vi "Line Output.vi"(8 "error in (no error)":errorcluster, 9 "position (0, 0)":cluster{"row":i8, "column":i8}, 10 "character codes":u8[](array[numeric])=[48, 49, 50, 51, 52, 53, 54, 55, 56, 57], 11 "cluster of private data in":T1={"FPGA VI Reference"=refnum, "device index"=0, "screen size"=enum."8x1", "font size"=enum."5x8", "auto wrap"=FALSE, "alignment"=enum."None", "number of line"=enum."2 lines", "shift 0"=0, "entry mode 0"=enum."increment & no shift", "shift 1"=0, "entry mode 1"=enum."increment & no shift"}) -> (0 "error out":errorcluster, 1 "current position":cluster{"row":i8, "column":i8}, 3 "cluster of private data out":T1={"FPGA VI Reference"=refnum, "device index"=0, "screen size"=enum."8x1", "font size"=enum."5x8", "auto wrap"=FALSE, "alignment"=enum."None", "number of line"=enum."2 lines", "shift 0"=0, "entry mode 0"=enum."increment & no shift", "shift 1"=0, "entry mode 1"=enum."increment & no shift"})   [LabVIEW 2017, in "HD44780.lvclass"]
uses:
  HD44780.lvclass
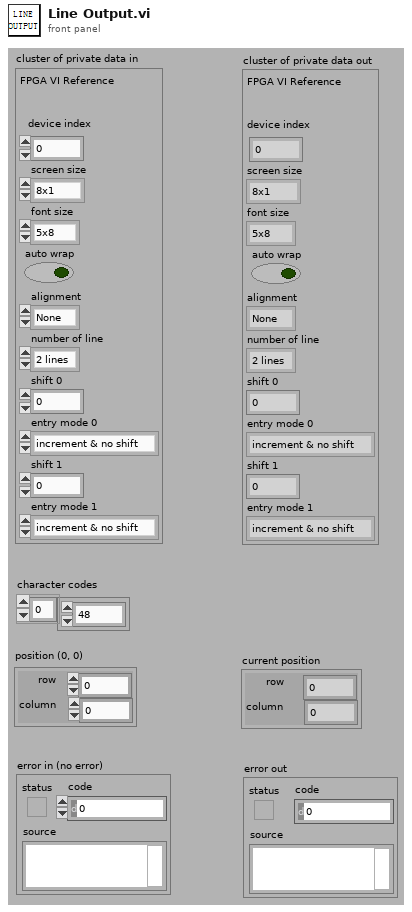
[diagram p1: front panel]
types:
  T1 = cluster{"FPGA VI Reference":refnum<k20>, "device index":i8, "screen size":enum8{"8x1", "8x2", "12x4", "16x1", "16x2", "16x4", "20x1", "20x2", "20x4", "24x1", "24x2", "40x2", "40x4"}, "font size":enum8{"5x8", "5x10"}, "auto wrap":bool, "alignment":enum16{"None", "Left", "Center", "Right"}, "number of line":enum8{"1 line", "2 lines"}, "shift 0":i8, "entry mode 0":enum8{"increment & no shift", "increment & shift", "decrement & no shift", "decrement & shift"}, "shift 1":i8, "entry mode 1":enum8{"increment & no shift", "increment & shift", "decrement & no shift", "decrement & shift"}}
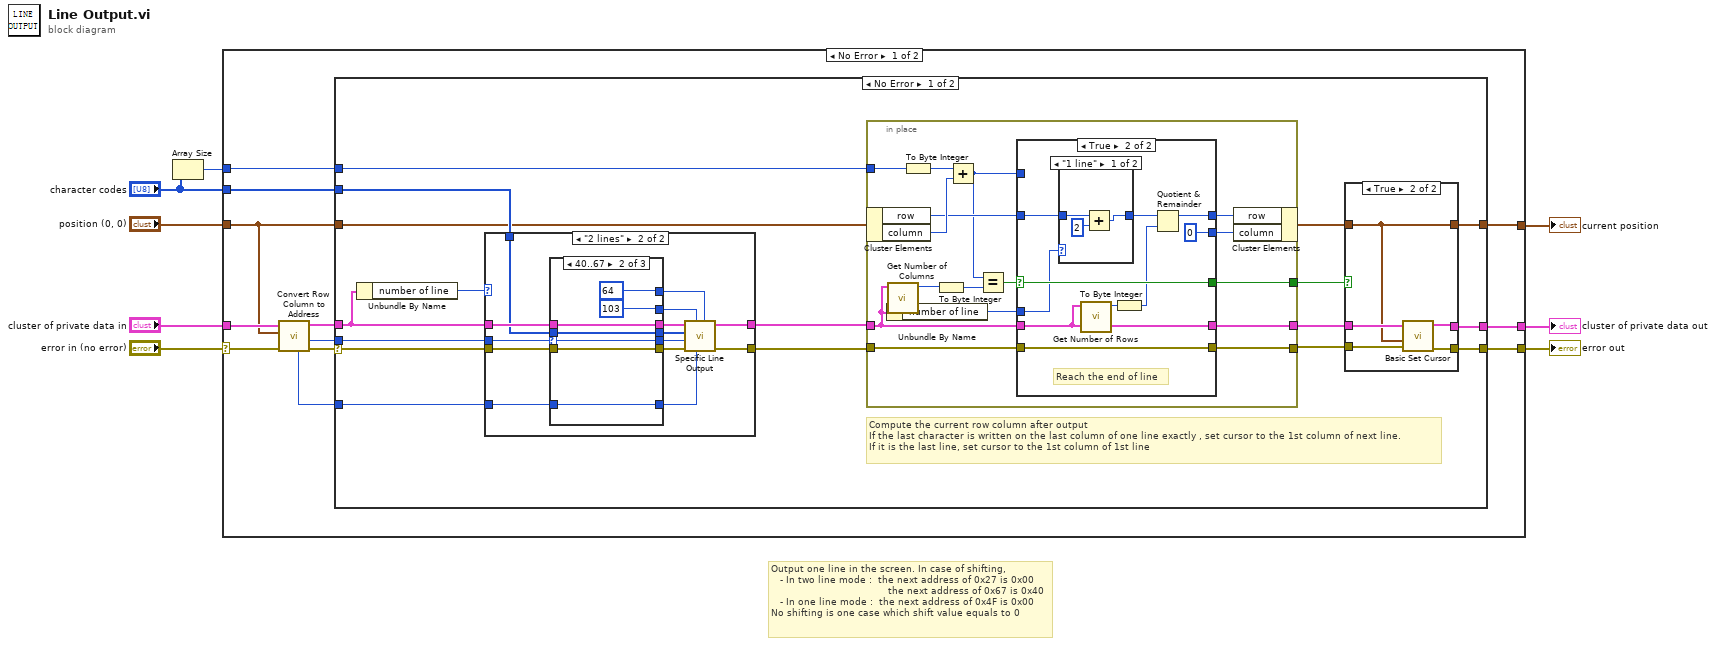
[diagram p0: block diagram]
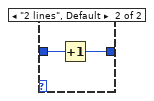
[diagram p4: hidden frame]
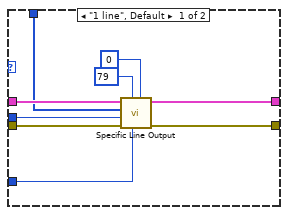
[diagram p5: hidden frame]
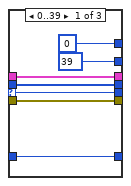
[diagram p6: hidden frame]
diagram:
  # "Output one line in the screen. In case of shifting,\n   - In two line mode :  the next address of 0x27 is 0x00\n                                       the next address of 0x67 is 0x40\n   - In one line mode :  the next address of 0x4F is 0x00\nNo shifting is one case which shift value equals to 0"
  n1 = Array Size(array="character codes") -> (size(s)=w5:i32)
  n2 = case shown="No Error" "error in (no error)" {
    selector: "error in (no error)" -> [w16 w129]
    tunnel: [w12 w129] -> w1
    tunnel: "character codes" -> [w19 _]
    tunnel: "position (0, 0)" -> [w14 w127]
    tunnel: "cluster of private data in" -> [w17 w128]
    tunnel: [w13 w128] -> w2
    tunnel: w5 -> [w15 _]
    tunnel: [w11 w127] -> w3
    frame No Error {
      n3 = call "Convert Row Column to Address.vi"("error in (no error)"=w16, "cursor position"=w14, "cluster of private data in"=w17) -> ("error out"=w9:errorcluster, "address"=w10:u8, "cluster of private data out"=w20:T1, "chip select"=w18:enum16{"1st chip", "2nd chip"})  [unwired: 5 in]
      n4 = case shown="No Error" w9 {
        selector: w9 -> [w21 w124]
        tunnel: w20 -> [w37 w125]
        tunnel: w19 -> [w35 _]
        tunnel: w18 -> [w34 _]
        tunnel: w15 -> [w31 _]
        tunnel: w14 -> [w30 w126]
        tunnel: [w29 w125] -> w13
        tunnel: [w28 w124] -> w12
        tunnel: [w27 w126] -> w11
        tunnel: w10 -> [w26 _]
        frame No Error {
          # "Compute the current row column after output\nIf the last character is written on the last column of one line exactly , set cursor to the 1st column of next line.\nIf it is the last line, set cursor to the 1st column of 1st line"
          n5 = Unbundle By Name(w37) -> ("number of line"=w36:enum8{"1 line", "2 lines"})
          n6 = case shown="\"2 lines\"" w36 {
            tunnel: w37 -> [w88 w104]
            tunnel: w35 -> [w87 w102]
            tunnel: w34 -> [w84 w101]
            tunnel: w26 -> [w86 w100]
            tunnel: w21 -> [w85 w103]
            tunnel: [w83 w96] -> w32
            tunnel: [w82 w97] -> w33
            frame "1 line", Default {
              n7 = call "Specific Line Output.vi"("turn over address"=u8 0, "chip select"=w84, "end address"=u8 79, "error in (no error)"=w85, "start address"=w86, "character codes"=w87, "cluster of private data in"=w88) -> ("error out"=w83:errorcluster, "cluster of private data out"=w82:T1)  [unwired: 3 in]
            }
            frame "2 lines" {
              n8 = case shown="40..67" w100 {
                selector: w100 -> [w105 w113 w119]
                tunnel: w104 -> [w109 w118 w123]
                tunnel: w103 -> [w107 w117 w120]
                tunnel: w102 -> [w108 w114 w122]
                tunnel: w101 -> [w106 w112 w121]
                tunnel: [w109 w118 w123] -> w99
                tunnel: [w107 w117 w120] -> w98
                tunnel: [u8 0 u8 64 _] -> w95
                tunnel: [u8 39 u8 103 _] -> w94
                tunnel: [w108 w114 w122] -> w93
                tunnel: [w105 w113 w119] -> w92
                tunnel: [w106 w112 w121] -> w91
                frame 0..39 {
                }
                frame 64..103 {
                }
                frame Default {
                }
              }
              n9 = call "Specific Line Output.vi"("turn over address"=w95, "chip select"=w91, "end address"=w94, "error in (no error)"=w98, "start address"=w92, "character codes"=w93, "cluster of private data in"=w99) -> ("error out"=w96:errorcluster, "cluster of private data out"=w97:T1)  [unwired: 3 in]
            }
          }
          n10 = in-place {
            in-place-border: w31 -> [w60]
            in-place-border: w33 -> [w47]
            in-place-border: w32 -> [w50]
            in-place-border: [w49] -> w24
            in-place-border: [w51] -> w23
            in-place-border: [w48] -> w25
            n11 = in-place-cluster #1(w30) -> ("row"=w56:i8, "column"=w61:i8)
            n12 = Unbundle By Name(w47) -> ("number of line"=w46:enum8{"1 line", "2 lines"})
            n13 = call "Get Number of Columns.vi"("cluster of private data in"=w47) -> ("column number"=w52:u8)  [unwired: 10 in]
            n14 = To Byte Integer(number=w60) -> (8bit integer=w59:i8)
            n15 = To Byte Integer(number=w52) -> (8bit integer=w58:i8)
            n16 = Add(x=w59, y=w61) -> (x+y=w54:i8)
            n17 = Equal?(x=w54, y=w58) -> (x = y?=w57:bool)
            n18 = case shown="True" w57 {
              selector: w57 -> [w62 w75]
              tunnel: w56 -> [w66 w72]
              tunnel: [w66 w67] -> w55
              tunnel: w54 -> [w65 _]
              tunnel: [w65 i8 0] -> w53
              tunnel: w47 -> [w64 w71]
              tunnel: [w64 w71] -> w51
              tunnel: w50 -> [w63 w74]
              tunnel: [w63 w74] -> w49
              tunnel: [w62 w75] -> w48
              tunnel: w46 -> [_ w73]
              frame False {
              }
              frame True {
                # "Reach the end of line"
                n19 = case shown="\"1 line\"" w73 {
                  tunnel: w72 -> [w79 w81]
                  tunnel: [w77 w80] -> w69
                  frame "1 line" {
                    n20 = Add(x=w79, y=i8 2) -> (x+y=w77:i8)
                  }
                  frame "2 lines", Default {
                    n21 = Increment(x=w81) -> (x+1=w80:i8)
                  }
                }
                n22 = call "Get Number of Rows.vi"("cluster of private data in"=w71) -> ("row number"=w70:u8)  [unwired: 10 in]
                n23 = To Byte Integer(number=w70) -> (8bit integer=w68:i8)
                n24 = Quotient & Remainder(x=w69, y=w68) -> (x-y*floor(x/y)=w67:i8)  [unwired: 1 out]
              }
            }
            n25 = in-place-cluster #1("row"=w55, "column"=w53) -> (w22:cluster{"row":i8, "column":i8})
          }
          n26 = case shown="True" w25 {
            tunnel: w24 -> [w38 w45]
            tunnel: w23 -> [w39 w44]
            tunnel: [w39 w43] -> w29
            tunnel: [w38 w42] -> w28
            tunnel: w22 -> [w40 w41]
            tunnel: [w40 w41] -> w27
            frame False {
            }
            frame True {
              n27 = call "Basic Set Cursor.vi"("error in (no error)"=w45, "position"=w41, "cluster of private data"=w44) -> ("error out"=w42:errorcluster, "cluster of private data out"=w43:T1)  [unwired: 6 in, 1 out]
            }
          }
        }
        frame Error {
        }
      }
    }
    frame Error {
    }
  }
  "current position" <- w3
  "error out" <- w1
  "cluster of private data out" <- w2
